vi "medidor.vi"() -> ()   [LabVIEW 2021]
doc: "This example will show how to create simple instrument drivers high level example for EXFO PM 1623 instruments.\n\nThis example performs the following actions:\n1:Select power meter channel\n2:Changing the absolute measurement display\n3:Select new operating wavelength\n4:Fetch operation for the stored value"
uses:
  <instrlib>/EXFO PM 1xxx Series/EXFO PM 1xxx Series.lvlib
panel:
  out "output":dbl
  in  "input":dbl=1.1 caption="x"
  out "Power":dbl caption="Power Measurement" format="%_6e"
  in  "Channel Select (1)":u8=1 min=1 max=2
  in  "Power Unit (0:DBM)":u16(ring) items=["DBM", "W"]
  # "(c) 2010 EXFO Inc.  ALL RIGHTS RESERVED."
  # "Instrument Readings"
  # "Trigger Controls"
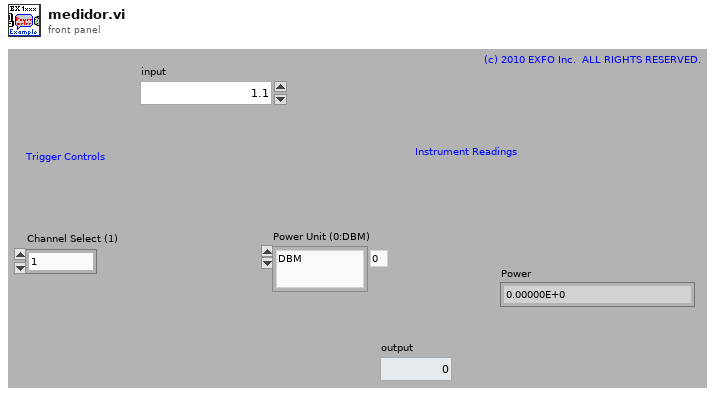
[diagram p1: front panel]
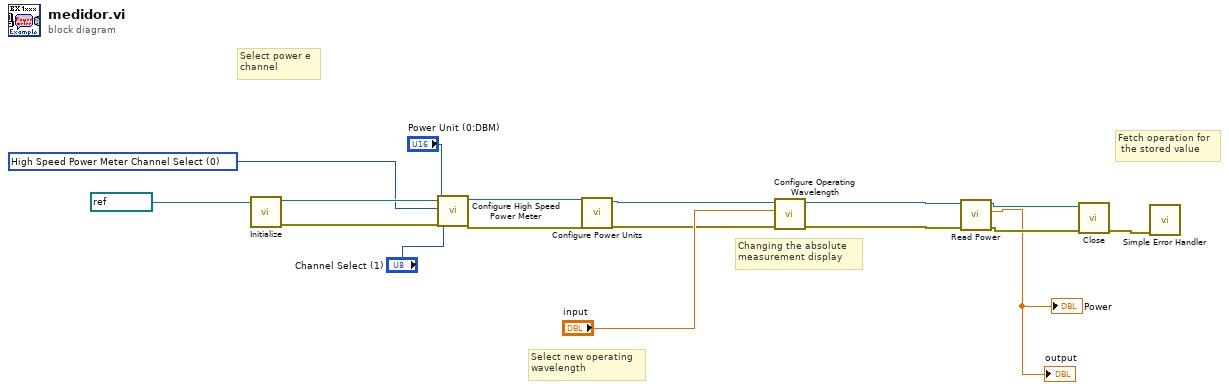
[diagram p0: block diagram]
diagram:
  w11 = u16 0 items=["High Speed Power Meter Channel Select", "High Speed Power Meter Power Range Auto", "High Speed Power Meter Power Range High", "High Speed Power Meter Power Range Low", "High Speed Power Meter Power Reference", "High Speed Power Meter Trace Points", "High Speed Power Meter Measurement Power Unit", "High Speed Power Meter Averaging Count", "High Speed Power Meter Auto Stop", "High Speed Power Meter High Sampling Rate", "High Speed Power Meter Low Sampling Rate"] ("High Speed Power Meter Command (0:High Speed Power Meter Channel Select)")
  # "Select new operating \nwavelength"
  # "Changing the absolute \nmeasurement display"
  # "Fetch operation for\n the stored value"
  # "Select power e \nchannel"
  n1 = call <instrlib>:"Initialize.vi"("VISA resource name"=refnum<visa-resource-name> "COM3") -> ("error out"=w15:errorcluster, "VISA resource name out"=w17:refnum<visa-resource-name>)  [unwired: 2 in, 7 out]
  n2 = call <instrlib>:"Configure High Speed Power Meter.vi"("VISA resource name"=w17, "High Speed Power Meter Command (0:High Speed Power Meter Channel Select)"=w11, "Measurement Power Unit (0:DB)"="Power Unit (0:DBM)", "error in (no error)"=w15, "Channel Select (1)"="Channel Select (1)") -> ("VISA resource name out"=w16:refnum<visa-resource-name>, "error out"=w14:errorcluster)  [unwired: 10 in, 11 out]
  n3 = call <instrlib>:"Configure Power Units.vi"("error in (no error)"=w14, "VISA resource name"=w16) -> ("error out"=w5:errorcluster, "VISA resource name out"=w6:refnum<visa-resource-name>)  [unwired: 1 in, 7 out]
  n4 = call <instrlib>:"Configure Operating Wavelength.vi"("error in (no error)"=w5, "Operating Wavelength(NM) (1310.12)"="input", "VISA resource name"=w6) -> ("error out"=w8:errorcluster, "VISA resource name out"=w9:refnum<visa-resource-name>)  [unwired: 7 out]
  n5 = call <instrlib>:"Read Power.vi"("error in (no error)"=w8, "VISA resource name"=w9) -> ("error out"=w3:errorcluster, "Power Measurement"=→"Power" →"output":dbl, "VISA resource name out"=w4:refnum<visa-resource-name>)  [unwired: 7 out]
  n6 = call <instrlib>:"Close.vi"("error in (no error)"=w3, "VISA resource name"=w4) -> ("error out"=w12:errorcluster)  [unwired: 9 out]
  n7 = call <vilib>:"Simple Error Handler.vi"("error in (no error)"=w12) -> ()  [unwired: 1 in, 8 out]
